vi "led sequential glowing using build array.vi"() -> ()   [LabVIEW 2018]
panel:
  out "1 10":bool
  out "1 9":bool
  out "1 8":bool
  out "1 7":bool
  out "1 6":bool
  out "1 5":bool
  out "1 4":bool
  out "1 3":bool
  out "1 2":bool
  out "1":bool
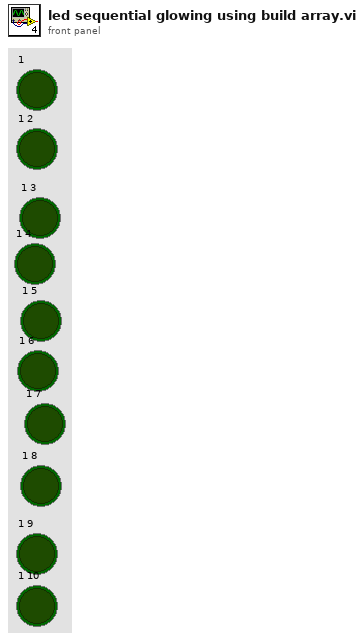
[diagram p1: front panel]
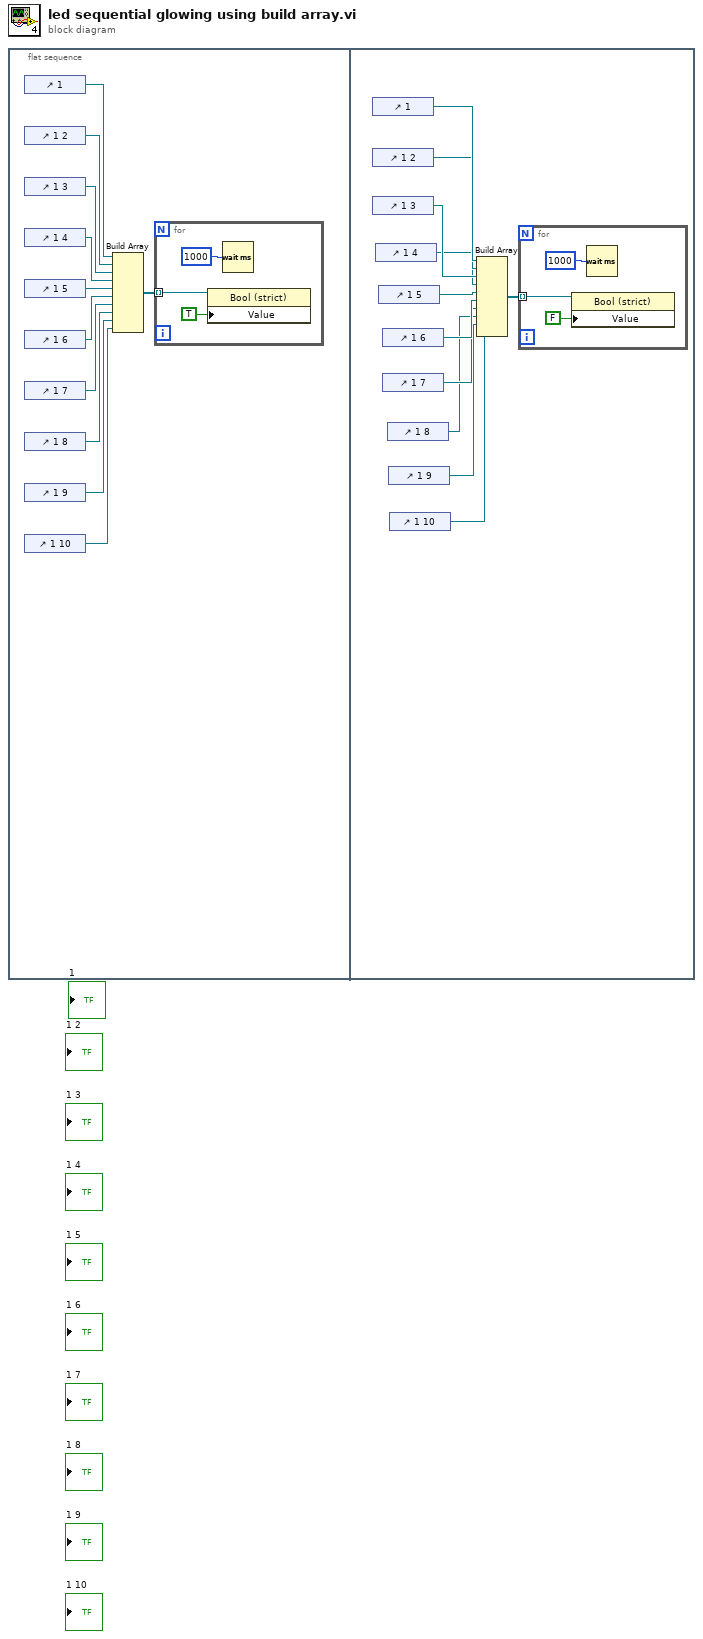
[diagram p0: block diagram]
diagram:
  n1 = flat-sequence {
    frame #0 {
      n2 = control-ref of="1"() -> (w11:refnum<vi>)
      n3 = control-ref of="1 2"() -> (w10:refnum<vi>)
      n4 = control-ref of="1 3"() -> (w9:refnum<vi>)
      n5 = control-ref of="1 4"() -> (w8:refnum<vi>)
      n6 = control-ref of="1 5"() -> (w7:refnum<vi>)
      n7 = control-ref of="1 6"() -> (w6:refnum<vi>)
      n8 = control-ref of="1 7"() -> (w5:refnum<vi>)
      n9 = control-ref of="1 8"() -> (w4:refnum<vi>)
      n10 = control-ref of="1 9"() -> (w3:refnum<vi>)
      n11 = control-ref of="1 10"() -> (w2:refnum<vi>)
      n12 = Build Array(w11, w10, w9, w8, w7, w6, w5, w4, w3, w2) -> (w1:refnum<vi>[])
      n13 = for {
        tunnel: w1 -> [w14] mode=indexing
        n14 = property class="Bool (strict)"(reference=w14, "Value"=TRUE) -> ()  [unwired: 1 in, 2 out]
        n15 = Wait (ms)(milliseconds to wait=u32 1000) -> ()  [unwired: 1 out]
      }
    }
    frame #1 {
      n16 = control-ref of="1"() -> (w24:refnum<vi>)
      n17 = control-ref of="1 2"() -> (w23:refnum<vi>)
      n18 = control-ref of="1 3"() -> (w22:refnum<vi>)
      n19 = control-ref of="1 4"() -> (w21:refnum<vi>)
      n20 = control-ref of="1 5"() -> (w20:refnum<vi>)
      n21 = control-ref of="1 6"() -> (w19:refnum<vi>)
      n22 = control-ref of="1 7"() -> (w18:refnum<vi>)
      n23 = control-ref of="1 8"() -> (w17:refnum<vi>)
      n24 = control-ref of="1 9"() -> (w16:refnum<vi>)
      n25 = control-ref of="1 10"() -> (w15:refnum<vi>)
      n26 = Build Array(w24, w23, w22, w21, w20, w19, w18, w17, w16, w15) -> (w25:refnum<vi>[])
      n27 = for {
        tunnel: w25 -> [w28] mode=indexing
        n28 = property class="Bool (strict)"(reference=w28, "Value"=FALSE) -> ()  [unwired: 1 in, 2 out]
        n29 = Wait (ms)(milliseconds to wait=u32 1000) -> ()  [unwired: 1 out]
      }
    }
  }
